vi "Read Output Angle.vi"(0 "VISA resource name":refnum<visa-resource-name>, 11 "error in (no error)":errorcluster) -> (4 "VISA resource name out":refnum<visa-resource-name>, 6 "Start Angle":dbl, 8 "End Angle":dbl, 15 "error out":errorcluster)   [LabVIEW 2016, in "APT 300XAC Series.lvlib"]
doc: "Reads the output angle (start and end angle) from the power source instrument.\n\nNote :\nProgram Mode : Step Parameter (Can be configured in every step individually).\nManual Mode : System Parameter ( Configuration affects all the memory)\nDC Mode : Not Supported"
uses:
  APT 300XAC Series.lvlib
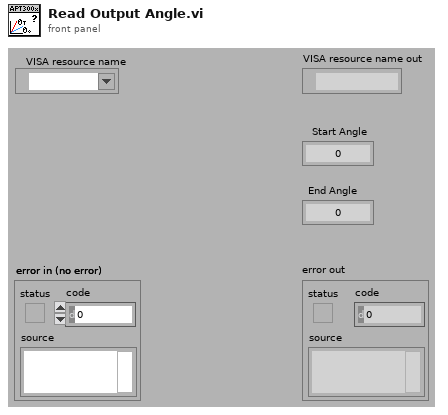
[diagram p1: front panel]
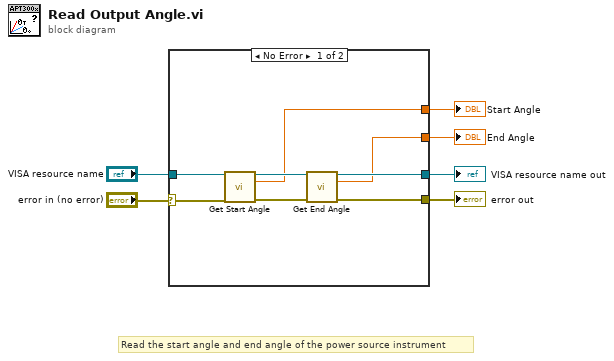
[diagram p0: block diagram]
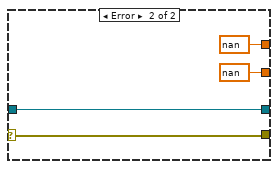
[diagram p2: hidden frame]
diagram:
  # "Read the start angle and end angle of the power source instrument"
  n1 = case shown="No Error" "error in (no error)" {
    selector: "error in (no error)" -> [w14 w17]
    tunnel: [w12 w17] -> w5
    tunnel: [w11 w18] -> w4
    tunnel: "VISA resource name" -> [w9 w18]
    tunnel: [w8 nan ("Voltage Low Limit")] -> w2
    tunnel: [w7 nan ("Voltage Low Limit")] -> w1
    frame No Error {
      n2 = call "Get Start Angle.vi"("VISA resource name"=w9, "error in (no error)"=w14) -> ("VISA resource name out"=w10:refnum<visa-resource-name>, "Start Angle"=w8:dbl, "error out"=w13:errorcluster)  [unwired: 11 in]
      n3 = call "Get End Angle.vi"("VISA resource name"=w10, "error in (no error)"=w13) -> ("VISA resource name out"=w11:refnum<visa-resource-name>, "End Angle"=w7:dbl, "error out"=w12:errorcluster)  [unwired: 11 in]
    }
    frame Error {
    }
  }
  "error out" <- w5
  "VISA resource name out" <- w4
  "Start Angle" <- w2
  "End Angle" <- w1
